vi "Excute.vi"(8 "error in (no error)":errorcluster, 11 "Cmd2 in":refnum<class "Cmd2.lvclass">) -> (0 "error out":errorcluster, 3 "Cmd2 out":refnum<class "Cmd2.lvclass">)   [LabVIEW 2014, in "Cmd2.lvclass"]
uses:
  Cmd2.lvclass
  Cmd2.lvclass/Cmd2.ctl
  Worker3/Worker3(receiver).lvclass
  Worker1/Worker1(receiver).lvclass
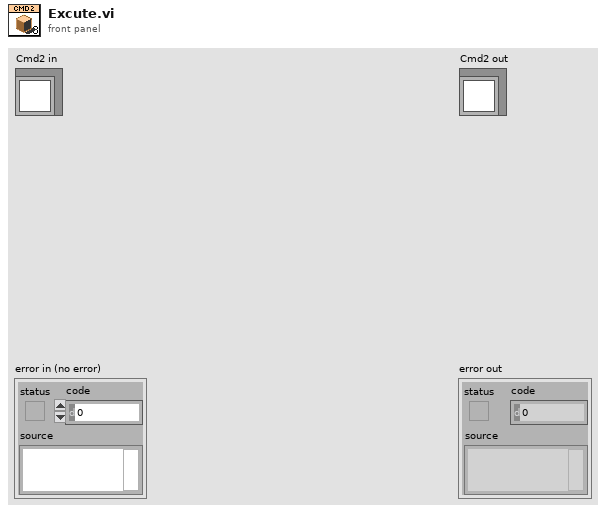
[diagram p1: front panel]
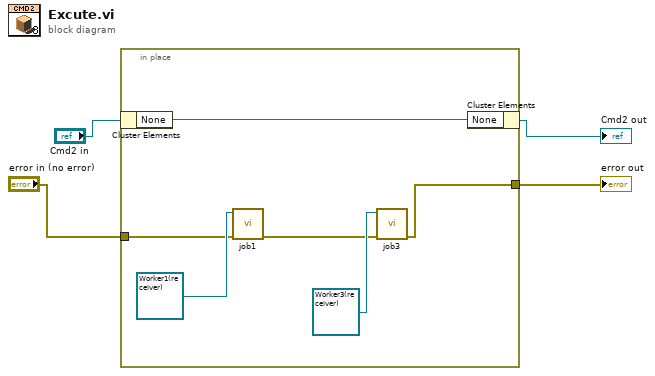
[diagram p0: block diagram]
diagram:
  n1 = in-place {
    in-place-border: "error in (no error)" -> [w6]
    in-place-border: [w5] -> w1
    n2 = in-place-cluster #1("Cmd2 in") -> ("None"=w10:bool)
    n3 = call "job1.vi"("error in (no error)"=w6, "Worker1(receiver) in"=refnum<class "Worker1(receiver).lvclass"> refnum ("Worker1(receiver).lvclass")) -> ("error out"=w7:errorcluster)  [unwired: 8 in, 1 out]
    n4 = call "job3.vi"("error in (no error)"=w7, "Worker3(receiver) in"=refnum<class "Worker3(receiver).lvclass"> refnum ("Worker3(receiver).lvclass")) -> ("error out"=w5:errorcluster)  [unwired: 8 in, 1 out]
    n5 = in-place-cluster #1("None"=w10) -> (→"Cmd2 out":refnum<class "Cmd2.lvclass">)
  }
  "error out" <- w1
